vi "Measure.vi"(8 "error in (no error)":errorcluster, 11 "RT_meas in":refnum<class "RT_meas.lvclass">) -> (0 "error out":errorcluster, 1 "Current Value":dbl, 2 "Result":dbl, 3 "RT_meas out":refnum<class "RT_meas.lvclass">)   [LabVIEW 2014, in "RT_meas.lvclass"]
uses:
  RT_meas.lvclass
  Abstract/Measurement/Measurement2D/Measurement2D.lvclass
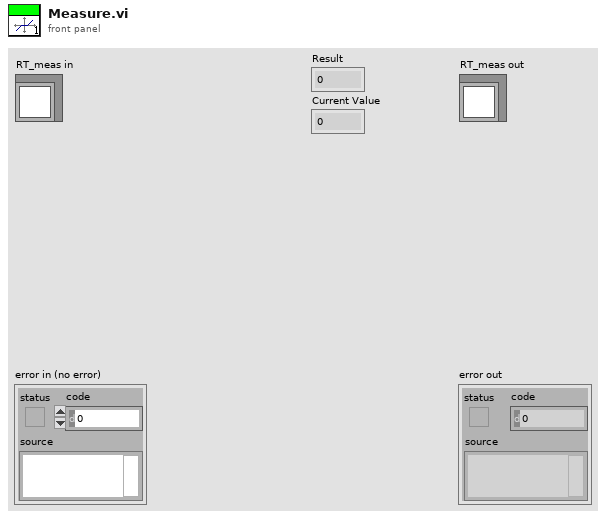
[diagram p1: front panel]
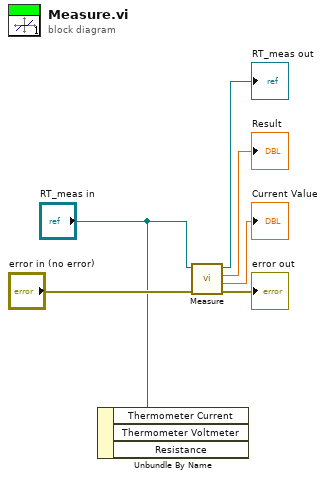
[diagram p0: block diagram]
diagram:
  n1 = Unbundle By Name("RT_meas in") -> ()  [unwired: 3 out]
  n2 = call-parent "Measure.vi"("error in (no error)"="error in (no error)", "Measurement2D in"="RT_meas in") -> ("error out"=→"error out":errorcluster, "Current Value"=→"Current Value":dbl, "Result"=→"Result":dbl, "Measurement2D out"=→"RT_meas out":refnum<class "RT_meas.lvclass">)  [unwired: 6 in]
